vi "{{Name}}.vi"(6 "Error in":errorcluster, 7 "{{Name}}":refnum<class "{{Name}}.lvclass">, 11 "{{Name}}":T1 {"MessageMetadata"."AbsoluteTime" format="%<%x %.3X>T"}) -> (3 "{{Name}}":T1 {"MessageMetadata"."AbsoluteTime" format="%<%x %.3X>T"}, 4 "Error out":errorcluster, 5 "{{Name}}":refnum<class "{{Name}}.lvclass">)   [LabVIEW 2020, in "_Template.lvlib" / "Templates.lvlib" / "{{Name}}Message.lvlib" / "{{Name}}.lvclass"]
uses:
  {{Name}}.lvclass
  Message.ctl
  {{Name}}Message.lvlib
  jettl/jettl/ActorRelation.ctl
  jettl/jettl/jettl.lvlib
  jettl/jettl/ActorLifetime.ctl
  jettl/jettl/MessageMetadata.ctl
panel:
  # "This front panel should not be manipulated."
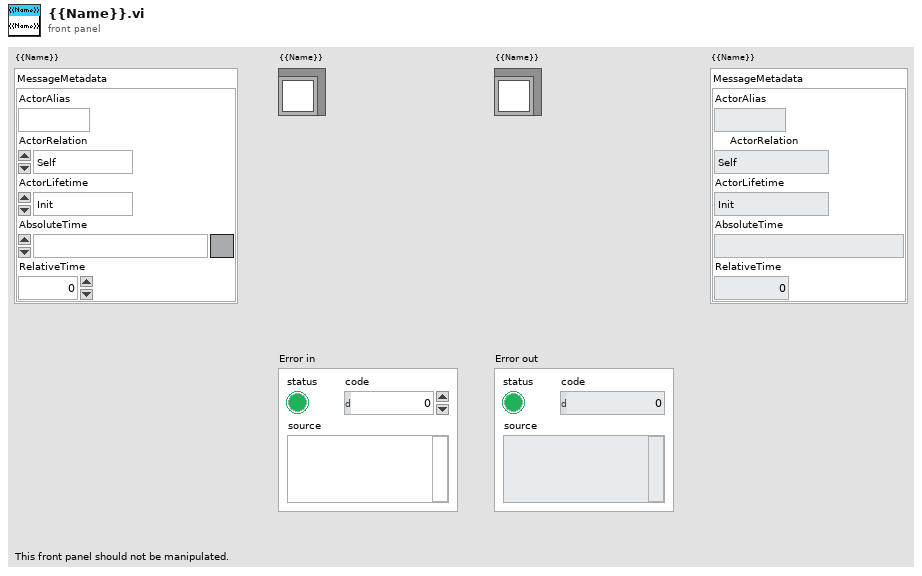
[diagram p1: front panel]
types:
  T1 = typedef "_Template.lvlib/Templates.lvlib/{{Name}}Message.lvlib/Message.ctl" = cluster{"MessageMetadata":T2}
  T2 = typedef "jettl.lvlib/MessageMetadata.ctl" = cluster{"ActorAlias":string, "ActorRelation":T3, "ActorLifetime":T4, "AbsoluteTime":timestamp, "RelativeTime":dbl}
  T3 = typedef "jettl.lvlib/ActorRelation.ctl" = enum16{"Self", "Actor"}
  T4 = typedef "jettl.lvlib/ActorLifetime.ctl" = enum16{"Init", "Spawn", "Setup", "Teardown Before Running", "Running", "Stop Called", "Stopping With Children", "Stopping Without Children", "Teardown After Running", "Stopped"}
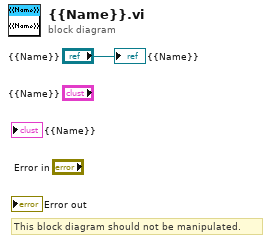
[diagram p0: block diagram]
diagram:
  # "This block diagram should not be manipulated."
  "{{Name}}" <- "{{Name}}"
